vi "Reset.vi"(11 "PID in":T1) -> (3 "PID out":T1)   [LabVIEW 2015, in "PID.lvlib"]
uses:
  PID.lvlib
  PID.ctl
  Anti-Windup Method.ctl
  Gains.ctl
  Output Range.ctl
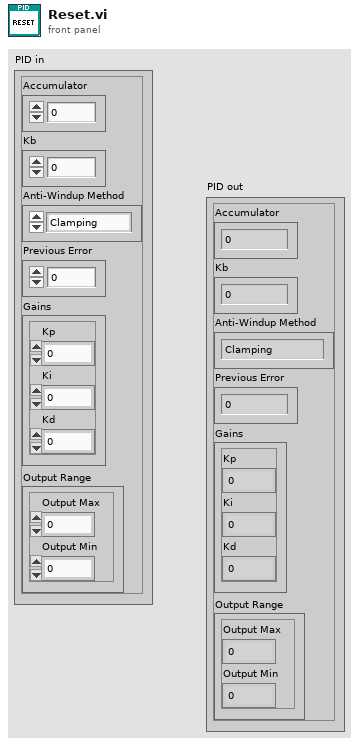
[diagram p1: front panel]
types:
  T1 = typedef "PID.lvlib/PID.ctl" = cluster{"Accumulator":dbl, "Kb":dbl, "Anti-Windup Method":T2, "Previous Error":dbl, "Gains":T3, "Output Range":T4}
  T2 = typedef "PID.lvlib/Anti-Windup Method.ctl" = enum16{"Clamping", "Back-Calculation", "None"}
  T3 = typedef "PID.lvlib/Gains.ctl" = cluster{"Kp":dbl, "Ki":dbl, "Kd":dbl}
  T4 = typedef "PID.lvlib/Output Range.ctl" = cluster{"Output Max":dbl, "Output Min":dbl}
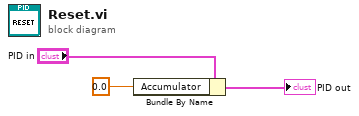
[diagram p0: block diagram]
diagram:
  n1 = Bundle By Name(cluster="PID in", "Accumulator"=0.0 ("Accumulated Error")) -> (→"PID out":T1)
